vi "Queue Comms Dequeue.vi"(8 "error in":errorcluster) -> (0 "error out":errorcluster, 3 "Data Out":T1={"Data"=variant, "Action"=enum."Error"})   [LabVIEW 2013, in "Contoller.lvlib"]
doc: "This VI dequeues data. Should be swapped\nif different comms method used."
uses:
  Contoller.lvlib
  Private Controls/Module Data Cluster.ctl
  Private Controls/Module Action.ctl
  Private Controls/Queue FG Action.ctl
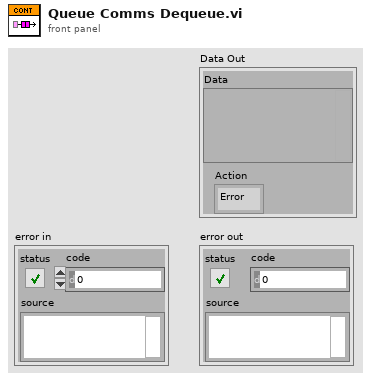
[diagram p1: front panel]
types:
  T1 = typedef "Contoller.lvlib/Module Data Cluster.ctl" = cluster{"Data":variant, "Action":T2}
  T2 = typedef "Contoller.lvlib/Module Action.ctl" = enum16{"Log In Init", "Fast Cash", "New transaction", "Withdrawal Init", "Recieve Keypad", "Deposit Finish", "Balance", "Withdrawal Approved", "Terminate", "Deposit Init", "Error", "Exit", "Init", "Log In Finish", "Cancel Transaction", "Withdrawal Failed", "Cash Removed"}
  T3 = typedef "Contoller.lvlib/Queue FG Action.ctl" = enum16{"Release", "Get", "Set"}
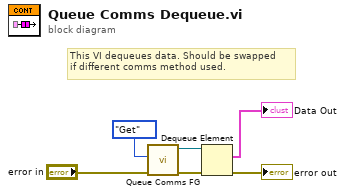
[diagram p0: block diagram]
diagram:
  # "This VI dequeues data. Should be swapped\nif different comms method used."
  n1 = call "Queue Comms FG.vi"("error in"="error in", "Action"=Queue_FG_Action."Get") -> ("error out"=w4:errorcluster, "Queue out"=w5:refnum<queue>)  [unwired: 8 in]
  n2 = Dequeue Element(queue=w5, error in (no error)=w4) -> (element=→"Data Out":T1, error out=→"error out":errorcluster)  [unwired: 1 in, 2 out]
